vi "Execute.vi"(8 "error in":errorcluster, 11 "BOOL STEP in":refnum<class "BOOL STEP.lvclass">) -> (0 "error out":errorcluster, 1 "Next Step?":bool, 2 "MSG":string, 3 "BOOL STEP out":refnum<class "BOOL STEP.lvclass">)   [LabVIEW 2014, in "BOOL STEP.lvlib" / "BOOL STEP.lvclass"]
uses:
  BOOL STEP.lvclass
  Send MSG STEP.lvlibp/Send MSG STEP.lvclass
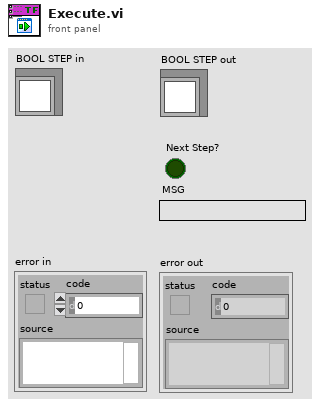
[diagram p1: front panel]
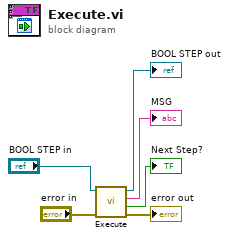
[diagram p0: block diagram]
diagram:
  n1 = call-parent "Execute.vi"("error in"="error in", "STEP in"="BOOL STEP in") -> ("error out"=→"error out":errorcluster, "Next Step?"=→"Next Step?":bool, "MSG"=→"MSG":string, "STEP out"=→"BOOL STEP out":refnum<class "BOOL STEP.lvclass">)  [unwired: 6 in]
